vi "Digitizer Scan Fetch Data.vi"(0 "instrument handle":refnum<k15>, 1 "Channel":string, 5 "Record":i32 format="%.0g", 7 "FirstPoint":i32 format="%.0g", 9 "LastPoint":i32 format="%.0g", 11 "error in (no error)":errorcluster {"code" format="%.0x"}, 12 "ValBufferSize":i32=2048) -> (4 "instrument handle out":refnum<k15>, 6 "Val":dbl[](array[numeric]) format="%.2p", 8 "ValActualSize":i32, 15 "error out":errorcluster {"code" format="%.0x"})   [LabVIEW 2020, in "Keysight DAQ970.lvlib"]
doc: "Returns the specified range of readings on the specified record for a channel."
uses:
  Keysight DAQ970.lvlib
  KtDAQ970.dll
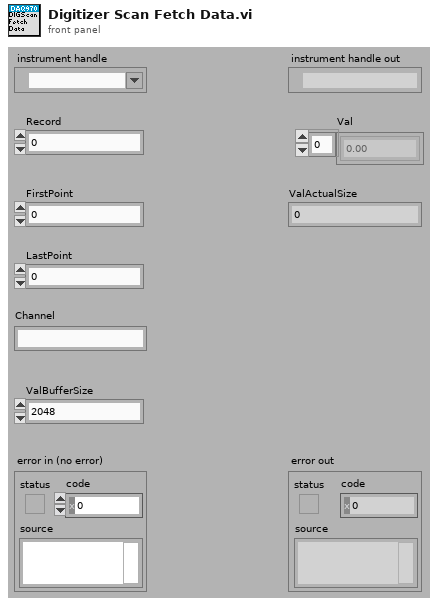
[diagram p1: front panel]
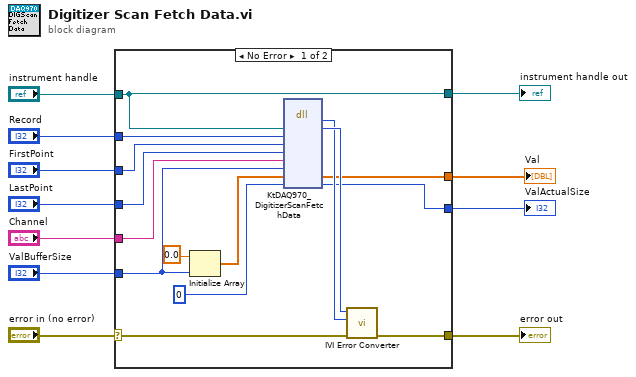
[diagram p0: block diagram]
diagram:
  n1 = case shown="No Error" "error in (no error)" {
    selector: "error in (no error)" -> [w24 w28]
    tunnel: [w23 w28] -> w11
    tunnel: "instrument handle" -> [w13 w27]
    tunnel: "Record" -> [w22 _]
    tunnel: "FirstPoint" -> [w21 _]
    tunnel: "LastPoint" -> [w20 _]
    tunnel: "Channel" -> [w19 _]
    tunnel: "ValBufferSize" -> [w12 _]
    tunnel: [w16 _] -> w3
    tunnel: [w14 _] -> w2
    tunnel: [w13 w27] -> w1
    frame No Error {
      n2 = Initialize Array(0.0 ("element"), w12) -> (w18:dbl[])
      n3 = dll-call lib="KtDAQ970**.dll" fn="KtDAQ970_DigitizerScanFetchData"("Vi"=w13, "Record"=w22, "FirstPoint"=w21, "LastPoint"=w20, "Channel"=w19, "ValBufferSize"=w12, "Val"=w18, "ValActualSize"=0) -> (w25:i32, "Vi"=w26:u32, "Val"=w16:dbl[], "ValActualSize"=w14:i32)  [unwired: 8 in, 2 out]
      n4 = call "IVI Error Converter.vi"("error in (no error)"=w24, "IVI error code (0)"=w25, "instrument handle"=w26) -> ("error out"=w23:errorcluster)  [unwired: 7 in, 1 out]
    }
    frame Error {
    }
  }
  "error out" <- w11
  "instrument handle out" <- w1
  "Val" <- w3
  "ValActualSize" <- w2
